vi "SSP - get value.vi"(8 "error in (no error)":errorcluster, 11 "JSON string":string) -> (0 "error out":errorcluster, 3 "value":string)   [LabVIEW 2020, in "ui-testing.lvlib"]
doc: "copyright: Thomas Zilliox©"
uses:
  ui-testing.lvlib
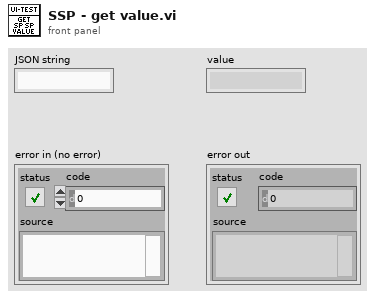
[diagram p1: front panel]
types:
  T1 = cluster{"control":string, "subpanel":string, "subsubpanel":string}
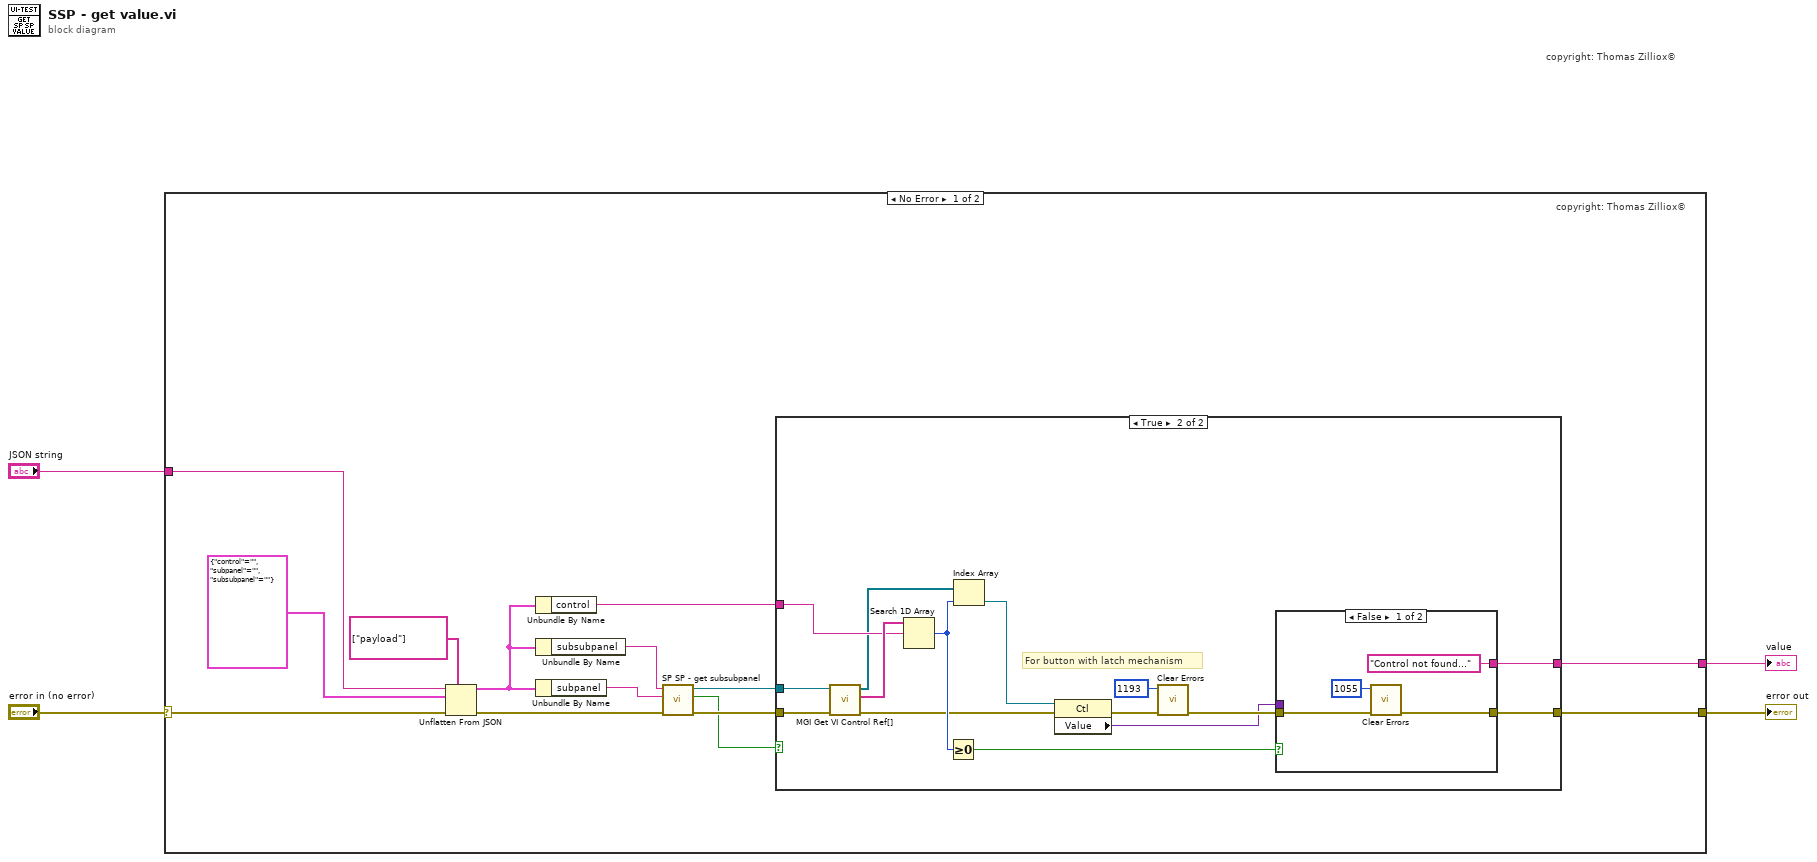
[diagram p0: block diagram]
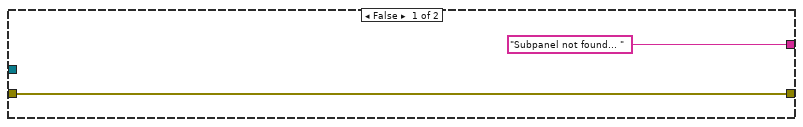
[diagram p2: hidden frame]
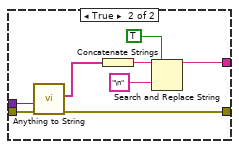
[diagram p3: hidden frame]
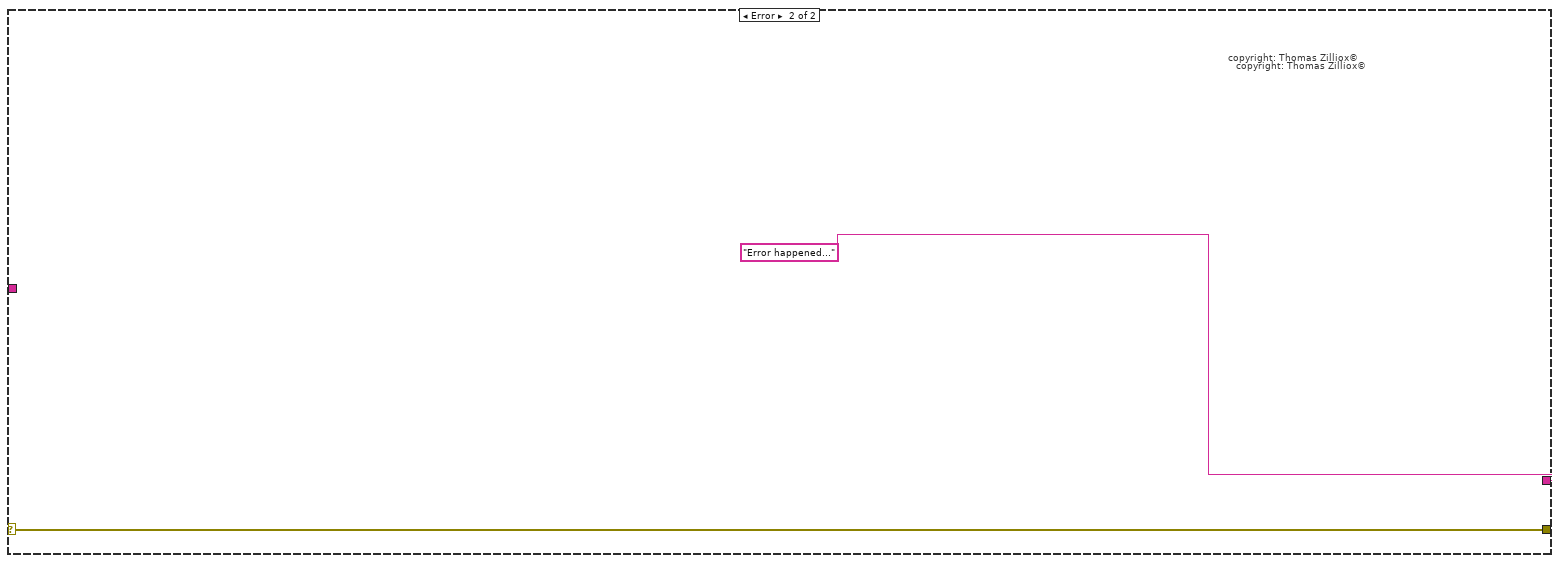
[diagram p4: hidden frame]
diagram:
  # "copyright: Thomas Zilliox©"
  n1 = case shown="No Error" "error in (no error)" {
    selector: "error in (no error)" -> [w14 w49]
    tunnel: "JSON string" -> [w16 _]
    tunnel: [w15 w49] -> w3
    tunnel: [w13 "Error happened..."] -> w1
    frame No Error {
      # "copyright: Thomas Zilliox©"
      n2 = Unflatten From JSON(path=string[] ["payload"], JSON string=w16, type and defaults=T1 {"control"="", "subpanel"="", "subsubpanel"=""}, error in (no error)=w14) -> (value=w12:T1, error out=w17:errorcluster)  [unwired: 3 in]
      n3 = Unbundle By Name(w12) -> ("control"=w10:string)
      n4 = Unbundle By Name(w12) -> ("subsubpanel"=w7:string)
      n5 = Unbundle By Name(w12) -> ("subpanel"=w8:string)
      n6 = call "SP SP - get subsubpanel.vi"("error in (no error)"=w17, "subpanel"=w8, "subsubpanel"=w7) -> ("error out"=w9:errorcluster, "SubSubPanel found"=w5:bool, "SubSubPanel VI"=w6:refnum<vi>)  [unwired: 5 in, 1 out]
      n7 = case shown="True" w5 {
        tunnel: [w20 w35] -> w15
        tunnel: w6 -> [_ w33]
        tunnel: w9 -> [w20 w32]
        tunnel: w10 -> [_ w30]
        tunnel: ["Subpanel not found... " ("result string") w34] -> w13
        frame False {
        }
        frame True {
          # "For button with latch mechanism"
          n8 = call <userlib>:"MGI Get VI Control Ref[].vi"("error in"=w32, "VI (Caller)"=w33) -> ("error out"=w27:errorcluster, "Control Label Chain[i]"=w31:string[], "Control[i]"=w29:refnum<vi>[])  [unwired: 6 in, 1 out]
          n9 = Search 1D Array(1D array=w31, element=w30) -> (index of element=w28:i32)  [unwired: 1 in]
          n10 = Greater Or Equal To 0?(x=w28) -> (x >= 0?=w21:bool)
          n11 = Index Array(array=w29, index=w28) -> (element=w22:refnum<vi>)
          n12 = property class="Ctl"(reference=w22, error in=w27) -> (error out=w26:errorcluster, "Value"=w23:variant)  [unwired: 1 out]
          n13 = call <vilib>:"Clear Errors.vi"("error in (no error)"=w26, "specific error code to clear (0: all)"=1193) -> ("error out"=w24:errorcluster)  [unwired: 4 in, 1 out]
          n14 = case shown="False" w21 {
            tunnel: w24 -> [w39 w47]
            tunnel: w23 -> [_ w46]
            tunnel: [w37 w45] -> w35
            tunnel: ["Control not found..." ("result string") w40] -> w34
            frame False {
              n15 = call <vilib>:"Clear Errors.vi"("error in (no error)"=w39, "specific error code to clear (0: all)"=1055) -> ("error out"=w37:errorcluster)  [unwired: 4 in, 1 out]
            }
            frame True {
              n16 = call <userlib>:"Anything to String.vi"("Error In"=w47, "Anything"=w46) -> ("Error Out"=w45:errorcluster, "Strings[]"=w41:string[])  [unwired: 7 in, 1 out]
              n17 = Concatenate Strings(w41) -> (w44:string)
              n18 = Search and Replace String(replace all?=TRUE ("replace all? (F)"), input string=w44, search string="\n") -> (result string=w40:string)  [unwired: 5 in, 3 out]
            }
          }
        }
      }
    }
    frame Error {
      # "copyright: Thomas Zilliox©"
      # "copyright: Thomas Zilliox©"
    }
  }
  "error out" <- w3
  "value" <- w1
